vi "Log to Clipboard.vi"(8 "error in (no error)":errorcluster, 11 "Log in":refnum<class "Log.lvclass">) -> (0 "error out":errorcluster, 3 "Log out":refnum<class "Log.lvclass">)   [LabVIEW 2015, in "AMS UI.lvlib" / "Log.lvclass"]
uses:
  Log.lvclass
  Log.lvclass/Log.ctl
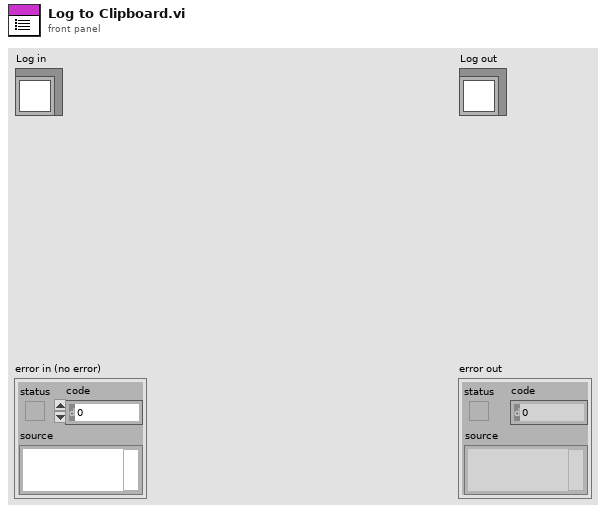
[diagram p1: front panel]
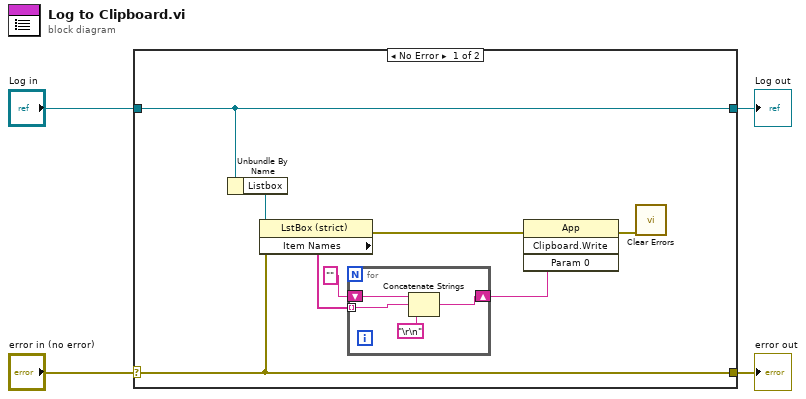
[diagram p0: block diagram]
diagram:
  n1 = case shown="No Error" "error in (no error)" {
    selector: "error in (no error)" -> [w5 w18]
    tunnel: [w5 w18] -> w3
    tunnel: [w11 w17] -> w1
    tunnel: "Log in" -> [w11 w17]
    frame No Error {
      n2 = Unbundle By Name(w11) -> ("Listbox"=w10:refnum<vi>)
      n3 = property on="Property Node" class="LstBox (strict)"(reference=w10, error in=w5) -> (error out=w12:errorcluster, "Item Names"=w9:string[])  [unwired: 1 out]
      n4 = for {
        tunnel: w9 -> [w16] mode=indexing
        shift-right: [w13] -> w7
        shift-left: "" -> [w15]
        n5 = Concatenate Strings(w15, w16, "\r\n") -> (w13:string)
      }
      n6 = invoke class="App" method="Clipboard.Write"(error in=w12, "Param 0"=w7) -> (error out=w6:errorcluster)  [unwired: 2 in, 3 out]
      n7 = call <vilib>:"Clear Errors.vi"("error in (no error)"=w6) -> ()  [unwired: 5 in, 2 out]
    }
    frame Error {
    }
  }
  "error out" <- w3
  "Log out" <- w1
